vi "solar_voy Pack (HDR).vi"(9 "HDR_GUID":string, 10 "HDR":T1, 11 "PACKET":T5 {"last_time" format="%<%H:%M:%S%3u %m/%d/%y>T"}) -> (2 "HDR LabVIEW Flattened Values":string[](array[string]), 3 "ITEMS":T2[](array[typedef]), 5 "ENDIAN":enum8{"BIG", "LITTLE"}(ring))   [LabVIEW 2018]
doc: "This returns the header values and updates the 'HDR_ID' and 'HDR_GUID'."
uses:
  solar_voy_def/solar_voy_def_ctl ITEM TYPE.ctl
  type/solar_type Item Type.ctl
  solar_voy_def/solar_voy_def_ctl ITEM.ctl
  solar_voy_def/solar_voy_def_ctl PACKET_ID.ctl
  solar_voy_def/solar_voy_def_ctl PACKET.ctl
  solar_voy_def/solar_voy_def_ctl HDR.ctl
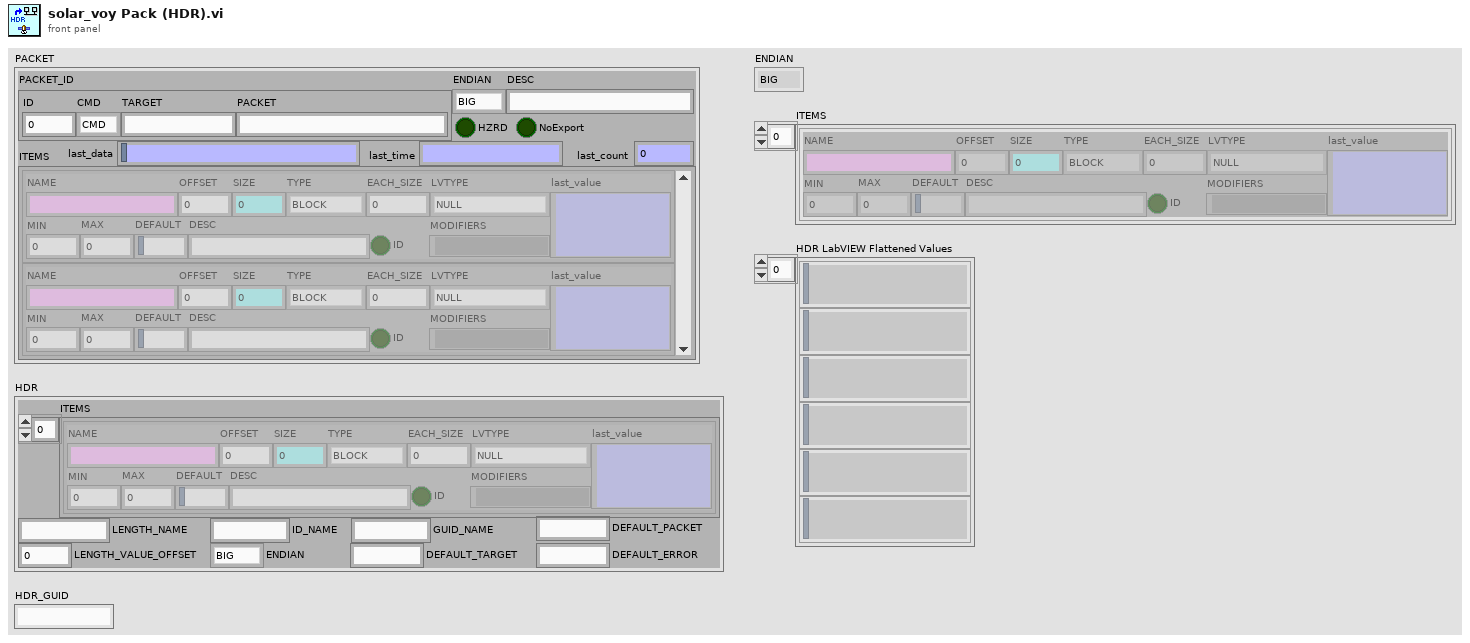
[diagram p1: front panel]
types:
  T1 = typedef "solar_voy_def_ctl HDR.ctl" = cluster{"ITEMS":T2[], "LENGTH_NAME":string, "LENGTH_VALUE_OFFSET":i32, "ID_NAME":string, "ENDIAN":enum8{"BIG", "LITTLE"}, "GUID_NAME":string, "DEFAULT_TARGET":string, "DEFAULT_PACKET":string, "DEFAULT_ERROR":string}
  T2 = typedef "solar_voy_def_ctl ITEM.ctl" = cluster{"NAME":string, "OFFSET":i32, "SIZE":i32, "TYPE":T3, "EACH_SIZE":i32, "LVTYPE":T4, "MIN":dbl, "MAX":dbl, "DEFAULT":string, "DESC":string, "ID":bool, "MODIFIERS":variant, "last_value":variant}
  T3 = typedef "solar_voy_def_ctl ITEM TYPE.ctl" = enum8{"BLOCK", "INT", "UINT", "FLOAT", "STRING"}
  T4 = typedef "solar_type Item Type.ctl" = enum16{"NULL", "UNKNOWN", "CLUSTER", "I8", "I16", "I32", "I64", "U8", "U16", "U32", "U64", "U8_ENUM", "U16_ENUM", "U32_ENUM", "SGL", "DBL", "BOOLEAN", "STRING", "PATH", "VISA", "TAG", "TIME", "I8_1D", "I16_1D", "I32_1D", "I64_1D", "U8_1D", "U16_1D", "U32_1D", "U64_1D", "U8_ENUM_1D", "U16_ENUM_1D", "U32_ENUM_1D", "SGL_1D", "DBL_1D", "BOOLEAN_1D", "STRING_1D", "PATH_1D", "VISA_1D", "TAG_1D", "TIME_1D", "I8_2D", "I16_2D", "I32_2D", "I64_2D", "U8_2D", "U16_2D", "U32_2D", "U64_2D", "U8_ENUM_2D", "U16_ENUM_2D", "U32_ENUM_2D", "SGL_2D", "DBL_2D", "BOOLEAN_2D", "STRING_2D", "PATH_2D", "VISA_2D", "TAG_2D", "TIME_2D"}
  T5 = typedef "solar_voy_def_ctl PACKET.ctl" = cluster{"PACKET_ID":T6, "ENDIAN":enum8{"BIG", "LITTLE"}, "DESC":string, "HZRD":bool, "ITEMS":T2[], "NoExport":bool, "last_time":timestamp, "last_count":u32, "last_data":string}
  T6 = typedef "solar_voy_def_ctl PACKET_ID.ctl" = cluster{"ID":u16, "CMD":enum8{"CMD", "TLM"}, "TARGET":string, "PACKET":string}
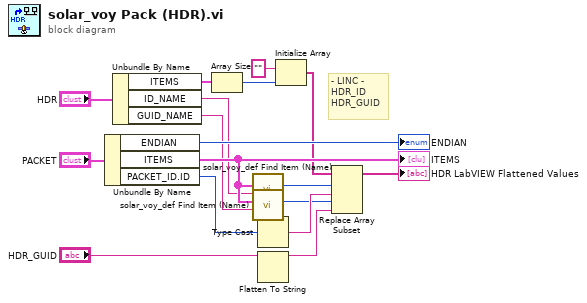
[diagram p0: block diagram]
diagram:
  # "- LINC -\nHDR_ID\nHDR_GUID"
  n1 = Unbundle By Name("PACKET") -> ("ENDIAN"=→"ENDIAN":enum8{"BIG", "LITTLE"}, "ITEMS"=w15:T2[], "PACKET_ID.ID"=w5:u16)
  "ITEMS" <- w15
  n2 = Unbundle By Name("HDR") -> ("ITEMS"=w10:T2[], "ID_NAME"=w11:string, "GUID_NAME"=w1:string)
  n3 = Array Size(array=w10) -> (size(s)=w9:i32)
  n4 = call "solar_voy_def Find Item (Name).vi"("ITEM_NAME"=w11, "ITEMS"=w15) -> ("Index"=w6:i32)  [unwired: 9 in]
  n5 = call "solar_voy_def Find Item (Name).vi"("ITEM_NAME"=w1, "ITEMS"=w15) -> ("Index"=w3:i32)  [unwired: 9 in]
  n6 = Type Cast(x=w5) -> (*(type *) &x=w4:string)  [unwired: 1 in]
  n7 = Flatten To String(anything="HDR_GUID") -> (data string=w17:string)  [unwired: 3 in, 2 out]
  n8 = Initialize Array("" ("data string"), w9) -> (w7:string[])
  n9 = Replace Array Subset(array=w7, new element #1=w4, index #1=w6, new element #2=w17, index #2=w3) -> (→"HDR LabVIEW Flattened Values":string[])
